vi "Translate.vi"(5 "To":string(combo)="ja", 8 "error in":errorcluster, 10 "テキスト":string, 11 "Handler":T1) -> (0 "error out":errorcluster, 2 "翻訳結果":string[](array[string]), 3 "Handler out":T1, 4 "body":string caption="Response body")   [LabVIEW 2015, in "LV_CloudTranslationAPI.lvlib"]
uses:
  LV_CloudTranslationAPI.lvlib
  Handler.ctl
  <vilib>/httpClient/ClientHandle.ctl
  <vilib>/httpClient/POSTBuffer.vi
  <vilib>/httpClient/LabVIEWHTTPClient.lvlib
panel:
  out "headers":string caption="Request header"
  out "headers":string caption="Response header"
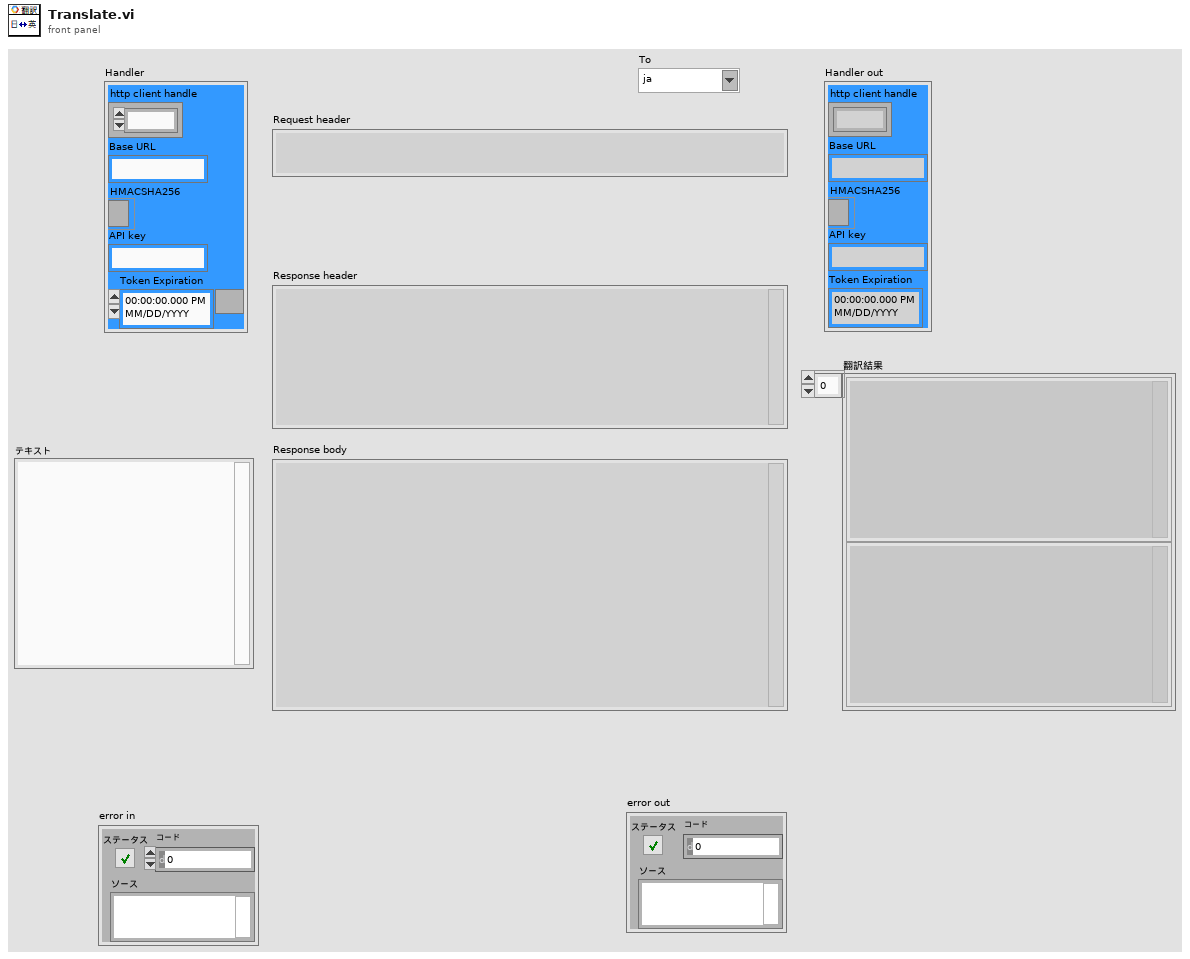
[diagram p1: front panel]
types:
  T1 = typedef "LV_CloudTranslationAPI.lvlib/Handler.ctl" = cluster{"http client handle":T2, "Base URL":string, "HMACSHA256":refnum<k24>, "API key":string, "Token Expiration ":timestamp}
  T2 = typedef "LabVIEWHTTPClient.lvlib/ClientHandle.ctl" = refnum<k1>
  T3 = cluster{"data":cluster{"translations":cluster{"detectedSourceLanguage":string, "translatedText":string}[]}}
  T4 = cluster{"detectedSourceLanguage":string, "translatedText":string}[]
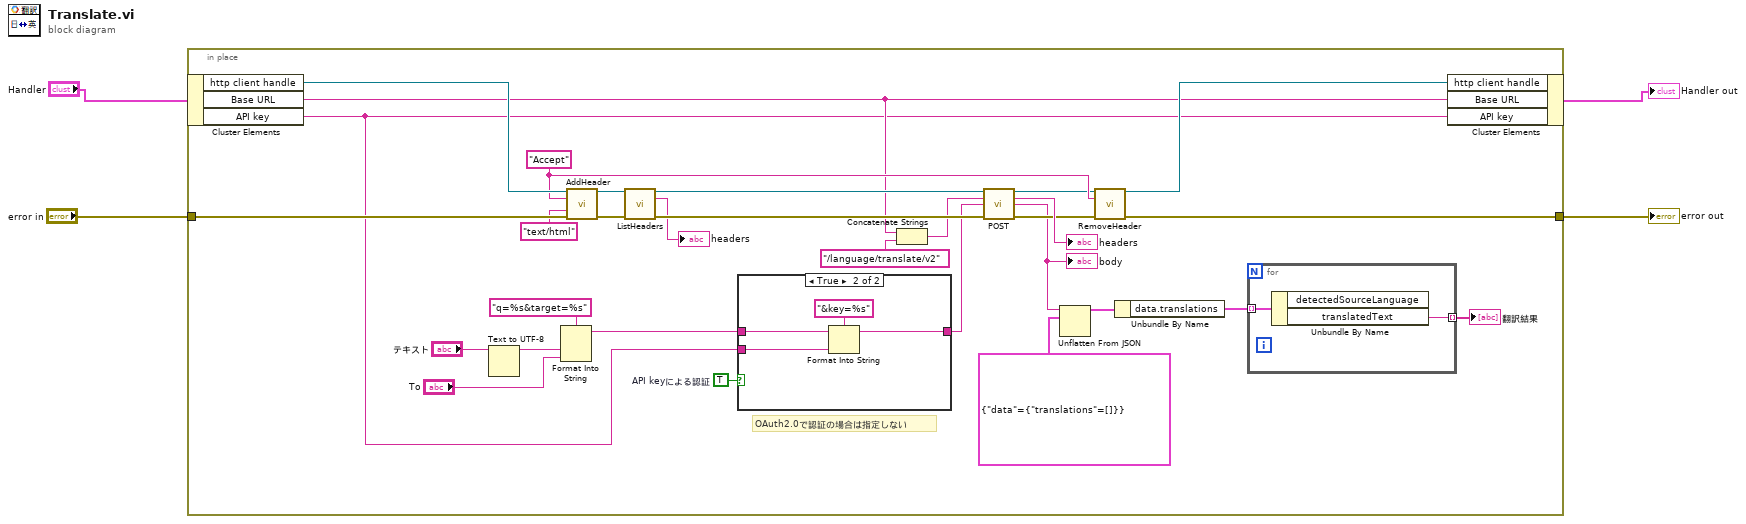
[diagram p0: block diagram]
diagram:
  n1 = in-place {
    in-place-border: "error in" -> [w34]
    in-place-border: [w22] -> w3
    w10 = TRUE  # API keyによる認証
    w26 = "Accept"
    # "OAuth2.0で認証の場合は指定しない"
    n2 = in-place-cluster #1("Handler") -> ("http client handle"=w32:T2, "Base URL"=w17:string, "API key"=w11:string)
    n3 = Text to UTF-8(11:"テキスト") -> (3:w18:string)  [unwired: 2 in, 1 out]
    n4 = Format Into String(format string="q=%s&target=%s" ("形式文字列"), w18, "To") -> (resulting string=w13:string)  [unwired: 2 in, 1 out]
    n5 = call <vilib>:"AddHeader.vi"("client handle"=w32, "header"=w26, "value"="text/html", "error in (no error)"=w34) -> ("client handle out"=w31:T2, "error out"=w30:errorcluster)  [unwired: 10 in]
    n6 = call <vilib>:"ListHeaders.vi"("client handle"=w31, "error in (no error)"=w30) -> ("client handle out"=w28:T2, "headers"=→"headers":string, "error out"=w29:errorcluster)  [unwired: 11 in]
    n7 = case shown="True" w10 {
      tunnel: w13 -> [w37 w41]
      tunnel: [w37 w40] -> w12
      tunnel: w11 -> [_ w38]
      frame False {
      }
      frame True {
        n8 = Format Into String(format string="&key=%s" ("形式文字列"), initial string=w41, w38) -> (resulting string=w40:string)  [unwired: 1 in, 1 out]
      }
    }
    n9 = Concatenate Strings(w17, "/language/translate/v2" ("文字列")) -> (w16:string)
    n10 = call-poly <vilib>:"POST.vi"("client handle"=w28, "url"=w16, "buffer"=w12, "error in (no error)"=w29) -> ("client handle out"=w25:T2, "headers"=→"headers":string, "body"=w9:string, "error out"=w23:errorcluster)  [unwired: 8 in]
    "body" <- w9
    n11 = Unflatten From JSON(JSON string=w9, type and defaults=T3 {"data"={"translations"=[]}} ("Root")) -> (value=w7:T3)  [unwired: 5 in, 1 out]
    n12 = call <vilib>:"RemoveHeader.vi"("client handle"=w25, "header"=w26, "error in (no error)"=w23) -> ("client handle out"=w24:T2, "error out"=w22:errorcluster)  [unwired: 11 in]
    n13 = Unbundle By Name(w7) -> ("data.translations"=w6:T4)
    n14 = for {
      tunnel: [w35] -> w5 mode=indexing
      tunnel: w6 -> [w36] mode=indexing
      n15 = Unbundle By Name(w36) -> ("translatedText"=w35:string)  [unwired: 1 out]
    }
    "翻訳結果" <- w5
    n16 = in-place-cluster #1("http client handle"=w24, "Base URL"=w17, "API key"=w11) -> (→"Handler out":T1)
  }
  "error out" <- w3
